vi "Normal Coefficient of Variation PDF.vi"(8 "Error In":errorcluster, 9 "n":i32, 10 "CV":dbl, 11 "x":dbl) -> (0 "Error Out":errorcluster, 3 "PDF (x)":dbl)   [LabVIEW 2021, in "Math.lvlib"]
uses:
  Math.lvlib
  <vilib>/gmath/NI_Gmath.lvlib
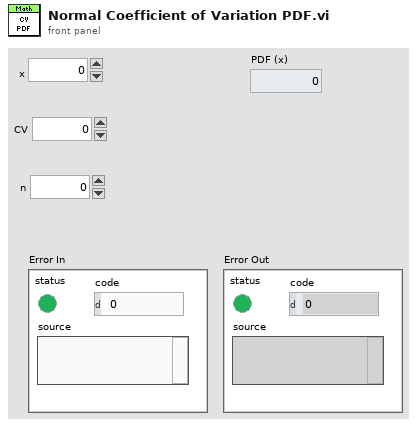
[diagram p1: front panel]
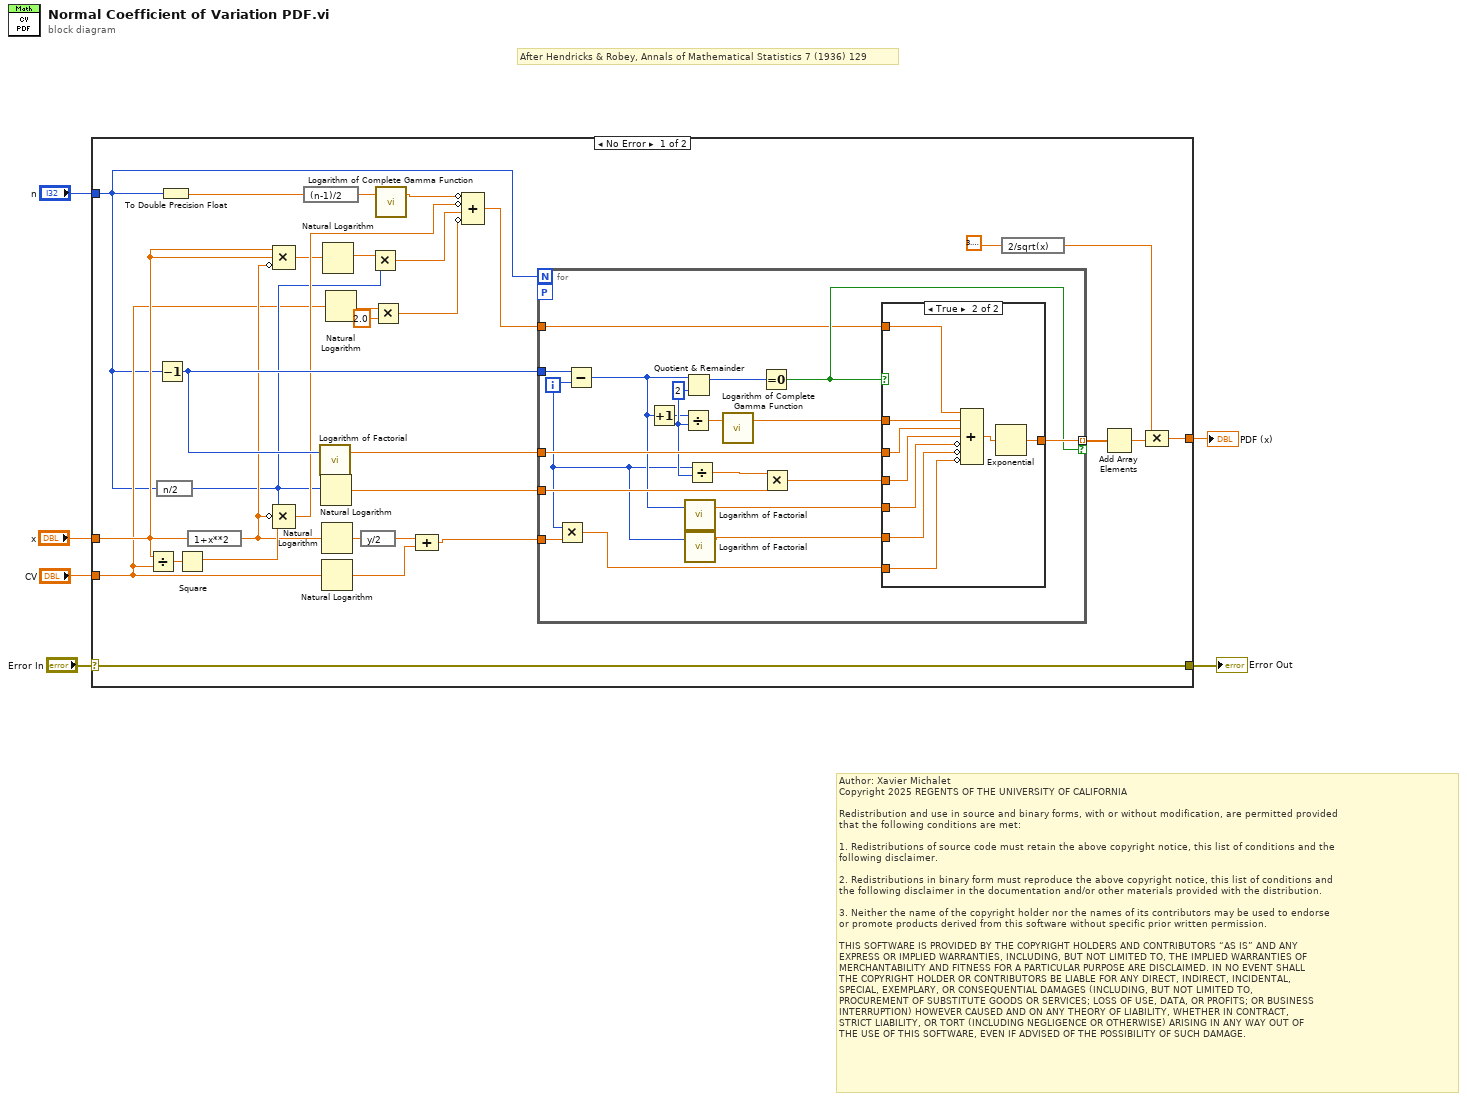
[diagram p0: block diagram]
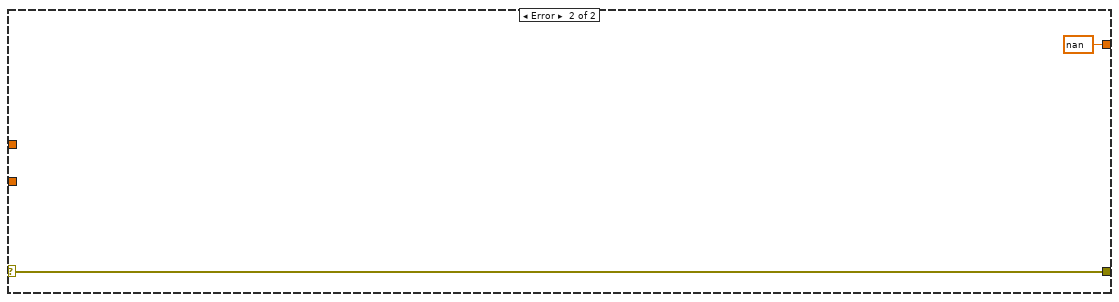
[diagram p3: hidden frame]
diagram:
  # "After Hendricks & Robey, Annals of Mathematical Statistics 7 (1936) 129"
  # "Author: Xavier Michalet\nCopyright 2025 REGENTS OF THE UNIVERSITY OF CALIFORNIA\n\nRedistribution and use in source and binary forms, with or without modification, are permitted provided\nthat the following conditions are met:\n\n1. Redistributions of source code must retain the above copyright notice, this list of conditions and the\nfollowing disclaimer.\n\n2. Redistributions in binary form must reproduce the above copyright notice, this list of conditions and\nthe following disclaimer in the documentation and/or other materials provided with the distribution.\n\n3. Neither the name of the copyright holder nor the names of its contributors may be used to endorse \nor promote products derived from this software without specific prior written permission.\n\nTHIS SOFTWARE IS PROVIDED BY THE COPYRIGHT HOLDERS AND CONTRIBUTORS “AS IS” AND ANY \nEXPRESS OR IMPLIED WARRANTIES, INCLUDING, BUT NOT LIMITED TO, THE IMPLIED WARRANTIES OF\nMERCHANTABILITY AND FITNESS FOR A PARTICULAR PURPOSE ARE DISCLAIMED. IN NO EVENT SHALL\nTHE COPYRIGHT HOLDER OR CONTRIBUTORS BE LIABLE FOR ANY DIRECT, INDIRECT, INCIDENTAL, \nSPECIAL, EXEMPLARY, OR CONSEQUENTIAL DAMAGES (INCLUDING, BUT NOT LIMITED TO, \nPROCUREMENT OF SUBSTITUTE GOODS OR SERVICES; LOSS OF USE, DATA, OR PROFITS; OR BUSINESS\nINTERRUPTION) HOWEVER CAUSED AND ON ANY THEORY OF LIABILITY, WHETHER IN CONTRACT, \nSTRICT LIABILITY, OR TORT (INCLUDING NEGLIGENCE OR OTHERWISE) ARISING IN ANY WAY OUT OF\nTHE USE OF THIS SOFTWARE, EVEN IF ADVISED OF THE POSSIBILITY OF SUCH DAMAGE."
  n1 = case shown="No Error" "Error In" {
    selector: "Error In" -> [w7 w67]
    tunnel: [w20 nan] -> w6
    tunnel: "x" -> [w18 _]
    tunnel: "CV" -> [w13 _]
    tunnel: "n" -> [w9 _]
    tunnel: [w7 w67] -> w1
    frame No Error {
      n2 = Divide(x=w18, y=w13) -> (x/y=w26:dbl)
      n3 = Decrement(x=w9) -> (x-1=w33:i32)
      n4 = expression code="n/2"(w9) -> (w15:i32)
      n5 = To Double Precision Float(number=w9) -> (double precision float=w29:dbl)
      n6 = Square(x=w26) -> (x^2=w25:dbl)
      n7 = expression code="1+x**2"(w18) -> (w19:dbl)
      n8 = Compound Arithmetic op=MULTIPLY(w18, w18, invert w19) -> (w17:dbl)
      n9 = Compound Arithmetic op=MULTIPLY(w15, invert w19, w25) -> (w24:dbl)
      n10 = expression code="(n-1)/2"(w29) -> (w28:dbl)
      n11 = call <vilib>:"Logarithm of Factorial.vi"("n"=w33) -> ("ln(n!)"=w32:dbl)  [unwired: 2 in]
      n12 = Natural Logarithm(1:w15) -> (0:w31:dbl)
      n13 = Natural Logarithm(1:w19) -> (0:w37:dbl)
      n14 = Natural Logarithm(1:w13) -> (0:w34:dbl)
      n15 = Natural Logarithm(1:w17) -> (0:w16:dbl)
      n16 = Natural Logarithm(1:w13) -> (0:w12:dbl)
      n17 = expression code="y/2"(w37) -> (w36:dbl)
      n18 = Multiply(x=w16, y=w15) -> (x*y=w14:dbl)
      n19 = Multiply(x=w12, y=2.0) -> (x*y=w10:dbl)
      n20 = call <vilib>:"Logarithm of Complete Gamma Function.vi"("x"=w28) -> ("ln(g(x))"=w27:dbl)  [unwired: 2 in]
      n21 = Compound Arithmetic op=ADD(w36, w34) -> (w35:dbl)
      n22 = Compound Arithmetic op=ADD(invert w27, invert w24, w14, invert w10) -> (w8:dbl)
      n23 = for {
        N: w9 -> [_]
        tunnel: w35 -> [w54]
        tunnel: w33 -> [w56]
        tunnel: w32 -> [w52]
        tunnel: w31 -> [w48]
        tunnel: [w41] -> w30 mode=indexing if=w40
        tunnel: w8 -> [w38]
        workers-P: _ -> [_]
        i -> [w44]
        w50 = 2 ("y")
        n24 = Multiply(x=w44, y=w54) -> (x*y=w42:dbl)
        n25 = Subtract(x=w56, y=w44) -> (x-y=w46:i32)
        n26 = Increment(x=w46) -> (x+1=w39:i32)
        n27 = Divide(x=w39, y=w50) -> (x/y=w53:dbl)
        n28 = Quotient & Remainder(x=w46, y=w50) -> (x-y*floor(x/y)=w55:i32)  [unwired: 1 out]
        n29 = call <vilib>:"Logarithm of Factorial.vi"("n"=w46) -> ("ln(n!)"=w45:dbl)  [unwired: 2 in]
        n30 = call <vilib>:"Logarithm of Factorial.vi"("n"=w44) -> ("ln(n!)"=w43:dbl)  [unwired: 2 in]
        n31 = Divide(x=w44, y=w50) -> (x/y=w49:dbl)
        n32 = call <vilib>:"Logarithm of Complete Gamma Function.vi"("x"=w53) -> ("ln(g(x))"=w51:dbl)  [unwired: 2 in]
        n33 = Equal To 0?(x=w55) -> (x = 0?=w40:bool)
        n34 = Multiply(x=w49, y=w48) -> (x*y=w47:dbl)
        n35 = case shown="True" w40 {
          tunnel: w52 -> [_ w64]
          tunnel: w51 -> [_ w65]
          tunnel: w47 -> [_ w63]
          tunnel: w45 -> [_ w62]
          tunnel: w43 -> [_ w61]
          tunnel: w42 -> [_ w60]
          tunnel: [_ w58] -> w41
          tunnel: w38 -> [_ w57]
          frame False {
          }
          frame True {
            n36 = Compound Arithmetic op=ADD(w57, w65, w64, w63, invert w62, invert w61, invert w60) -> (w59:dbl)
            n37 = Exponential(1:w59) -> (0:w58:dbl)
          }
        }
      }
      n38 = expression code="2/sqrt(x)"(3.141592653589793) -> (w22:dbl)
      n39 = Add Array Elements(numeric array=w30) -> (sum=w21:dbl)
      n40 = Compound Arithmetic op=MULTIPLY(w22, w21) -> (w20:dbl)
    }
    frame Error {
    }
  }
  "Error Out" <- w1
  "PDF (x)" <- w6
